vi "Set Trigger Settings.vi"(8 "error in (no error)":errorcluster, 10 "Trigger Settings":T1, 11 "TLCamera reference":refnum<k24>) -> (0 "error out":errorcluster, 3 "TLCamera reference out":refnum<k24>)   [LabVIEW 2015]
uses:
  C:/code/Host/Installer/Scientific Camera Interfaces/LabVIEW/64_bit/Library_X64/Thorlabs.TSI.TLCameraInterfaces.dll
  64_bit/Library_X64/Thorlabs.TSI.TLCameraInterfaces.dll
  Controls/Trigger Modes.ctl
  Controls/Trigger Polarity.ctl
  Controls/Trigger Settings.ctl
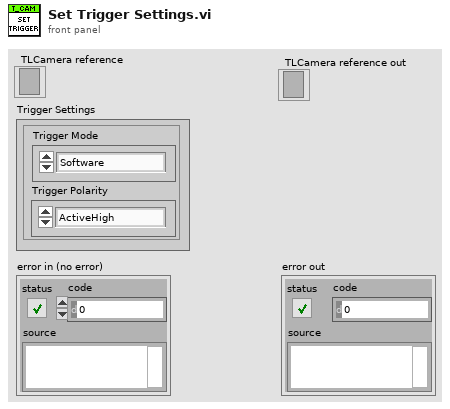
[diagram p1: front panel]
types:
  T1 = typedef "Trigger Settings.ctl" = cluster{"Trigger Mode":T2, "Trigger Polarity":T3}
  T2 = typedef "Trigger Modes.ctl" = enum16{"Software", "Hardware Standard", "Bulb(PDX) Mode"}
  T3 = typedef "Trigger Polarity.ctl" = enum32{"ActiveHigh", "ActiveLow"}
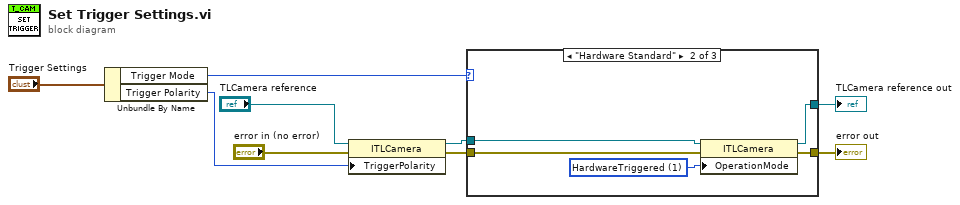
[diagram p0: block diagram]
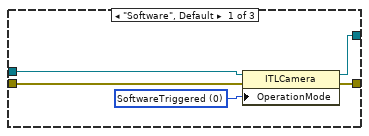
[diagram p2: hidden frame]
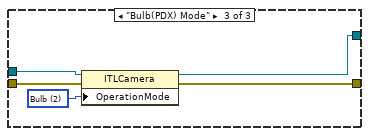
[diagram p3: hidden frame]
diagram:
  n1 = Unbundle By Name("Trigger Settings") -> ("Trigger Mode"=w7:T2, "Trigger Polarity"=w1:T3)
  n2 = property class="ITLCamera"(reference="TLCamera reference", error in="error in (no error)", "TriggerPolarity"=w1) -> (reference out=w6:refnum<k24>, error out=w5:errorcluster)
  n3 = case shown="\"Hardware Standard\"" w7 {
    tunnel: w6 -> [w14 w19 w24]
    tunnel: w5 -> [w13 w18 w23]
    tunnel: [w12 w17 w22] -> w4
    tunnel: [w11 w16 w21] -> w3
    frame "Software", Default {
      w10 = 0 items=["SoftwareTriggered", "HardwareTriggered", "Bulb", "Reserved1", "Reserved2"] ("OperationMode")
      n4 = property class="ITLCamera"(reference=w14, error in=w13, "OperationMode"=w10) -> (reference out=w12:refnum<k24>, error out=w11:errorcluster)
    }
    frame "Hardware Standard" {
      w15 = 1 items=["SoftwareTriggered", "HardwareTriggered", "Bulb", "Reserved1", "Reserved2"] ("OperationMode")
      n5 = property class="ITLCamera"(reference=w19, error in=w18, "OperationMode"=w15) -> (reference out=w17:refnum<k24>, error out=w16:errorcluster)
    }
    frame "Bulb(PDX) Mode" {
      w20 = 2 items=["SoftwareTriggered", "HardwareTriggered", "Bulb", "Reserved1", "Reserved2"] ("OperationMode")
      n6 = property class="ITLCamera"(reference=w24, error in=w23, "OperationMode"=w20) -> (reference out=w22:refnum<k24>, error out=w21:errorcluster)
    }
  }
  "error out" <- w3
  "TLCamera reference out" <- w4
